vi "Write_TextMark.vi"(1 "text":string, 2 "TextMark in":T1, 5 "type":i32) -> (7 "TextMark out":T1)   [LabVIEW 2016]
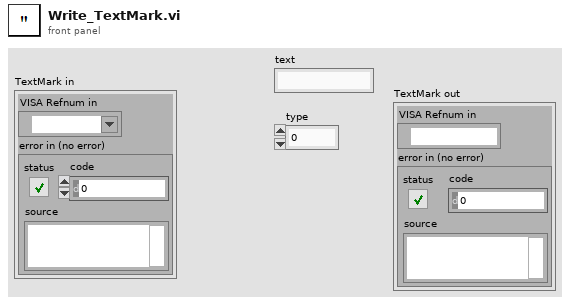
[diagram p1: front panel]
types:
  T1 = cluster{"VISA Refnum in":refnum<visa-resource-name>, "error in (no error)":errorcluster}
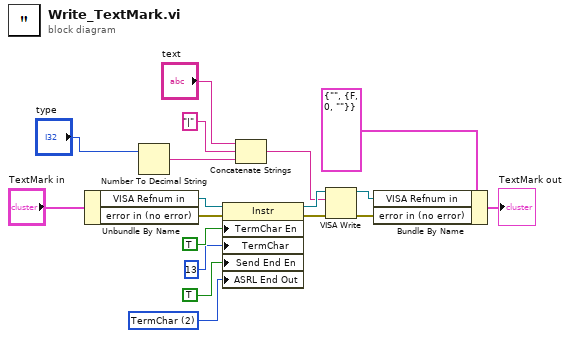
[diagram p0: block diagram]
diagram:
  w18 = u16 2 items=["None", "Last Bit", "TermChar", "Break"] ("Serial Settings:End Mode for Writes")
  n1 = Unbundle By Name("TextMark in") -> ("VISA Refnum in"=w6:refnum<visa-resource-name>, "error in (no error)"=w5:errorcluster)
  n2 = Number To Decimal String(number="type") -> (decimal integer string=w10:string)  [unwired: 1 in]
  n3 = property class="Instr"(reference=w6, error in=w5, "TermChar En"=TRUE ("Message Based Settings:Termination Character Enable"), "TermChar"=u8 13 ("Message Based Settings:Termination Character"), "Send End En"=TRUE ("Message Based Settings:Send End Enable"), "ASRL End Out"=w18) -> (reference out=w13:refnum<visa-resource-name>, error out=w14:errorcluster)
  n4 = Concatenate Strings("text", "|" ("string"), w10) -> (w12:string)
  n5 = VISA Write(VISA resource name=w13, write buffer=w12, error in (no error)=w14) -> (VISA resource name out=w3:refnum<visa-resource-name>, error out=w2:errorcluster)  [unwired: 1 out]
  n6 = Bundle By Name(cluster=T1 {"VISA Refnum in"="", "error in (no error)"={"status"=FALSE, "code"=0, "source"=""}} ("TextMark out"), "VISA Refnum in"=w3, "error in (no error)"=w2) -> (→"TextMark out":T1)
